vi "GOMDBTS2048 async Get Progress.vi"(8 "error in (no error)":errorcluster, 11 "handle":i32) -> (0 "error out":errorcluster, 1 "function return":i32, 2 "progress":i32, 3 "finished":bool)   [LabVIEW 2015, in "GOMDBTS2048.lvlib"]
doc: "GOBTS2048DLL int __stdcall GOMDBTS2048_asyncGetProgress(int handle, bool* finished, int* progress);"
uses:
  GOMDBTS2048.lvlib
  runtime/GOMDBTS2048.dll
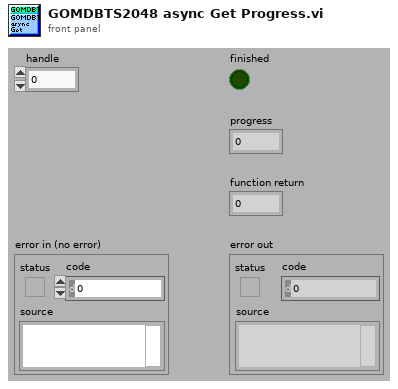
[diagram p1: front panel]
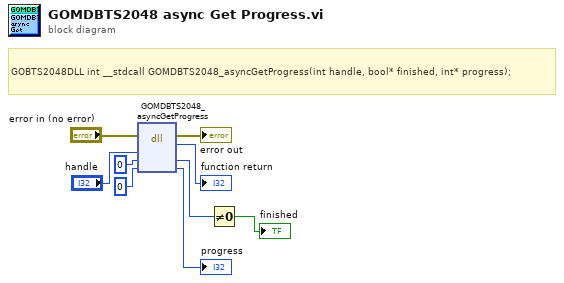
[diagram p0: block diagram]
diagram:
  # "GOBTS2048DLL int __stdcall GOMDBTS2048_asyncGetProgress(int handle, bool* finished, int* progress);"
  n1 = dll-call lib="C:/Users/rkoch/Documents/GO_Library/runtime/GOMDBTS2048.*" fn="GOMDBTS2048_asyncGetProgress"(error in="error in (no error)", "handle"="handle", "finished"=u8 0, "progress"=0) -> (error out=→"error out":errorcluster, →"function return":i32, "finished"=w5:u8, "progress"=→"progress":i32)  [unwired: 3 in, 1 out]
  n2 = Not Equal To 0?(x=w5) -> (x != 0?=→"finished":bool)
